vi "start_photon_stream.vi"(8 "error in (no error)":errorcluster, 11 "detector in":refnum<class "detector.lvclass">) -> (0 "error out":errorcluster, 3 "detector out":refnum<class "detector.lvclass">)   [LabVIEW 2015, in "detector.lvclass"]
uses:
  detector.lvclass
  detector.lvclass/detector.ctl
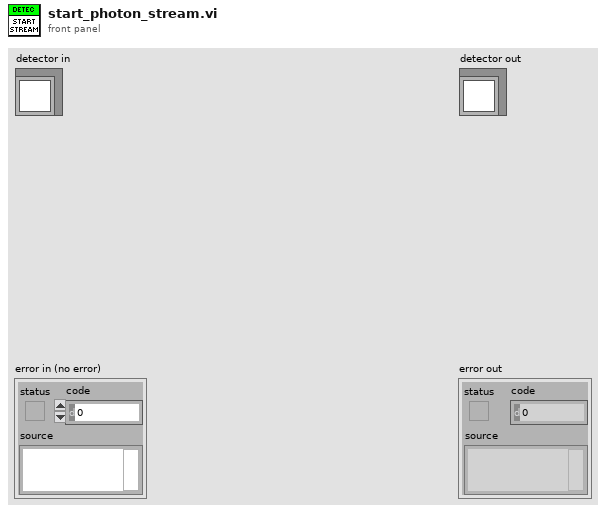
[diagram p1: front panel]
types:
  T1 = cluster{"stream":u64[], "channel":u8[], "sync":u64[], bool}
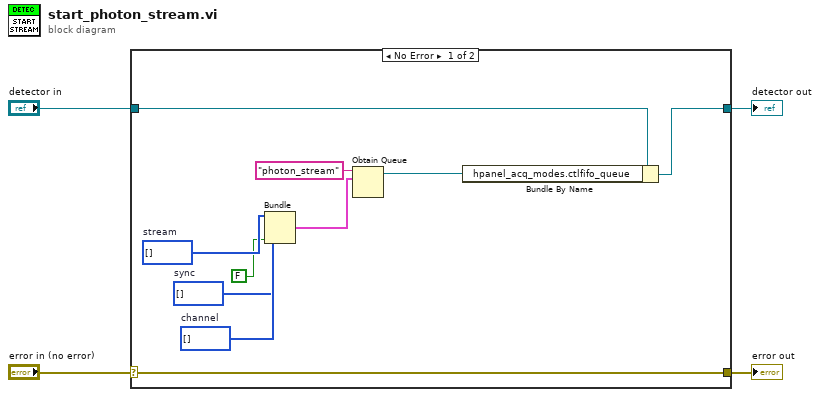
[diagram p0: block diagram]
diagram:
  n1 = case shown="No Error" "error in (no error)" {
    selector: "error in (no error)" -> [w14 w16]
    tunnel: [w14 w16] -> w3
    tunnel: [w5 w15] -> w1
    tunnel: "detector in" -> [w6 w15]
    frame No Error {
      w11 = u8[] []  # channel
      w10 = u64[] []  # sync
      w12 = u64[] []  # stream
      n2 = Bundle("stream"=w12, "channel"=w11, "sync"=w10, FALSE) -> (w9:T1)  [unwired: 1 in]
      n3 = Obtain Queue(name (unnamed)="photon_stream", element data type=w9) -> (queue out=w7:refnum<queue>)  [unwired: 3 in, 2 out]
      n4 = Bundle By Name(cluster=w6, "hpanel_acq_modes.ctlfifo_queue"=w7) -> (w5:refnum<class "detector.lvclass">)
    }
    frame Error {
    }
  }
  "error out" <- w3
  "detector out" <- w1
